vi "CollectData.vi"(7 "LabVIEW Web Service Request":refnum<class "Web Request.lvclass">) -> ()   [LabVIEW 2017]
uses:
  <vilib>/wsapi/Web Request.lvclass
  <vilib>/rvi/interface/nirviOpenFPGA/nirviOpenFPGA.xnode
  <vilib>/rvi/interface/nirviCloseFPGA/nirviCloseFPGA.xnode
  <vilib>/FPGAPlugInAG/Dynamic/niLvFpga_Close_Dynamic.vi
  <vilib>/rvi/interface/nirviReadWriteControl/nirviReadWriteControl.xnode
  NiFpgaLv.dll
  <vilib>/Utility/error.llb/Error Cluster From Error Code.vi
  <vilib>/rvi/interface/Simulation/niFpgaSimulationCallBeginRW.vi
  <vilib>/rvi/errors/niLvFpgaAdjustHostInterfaceError.vi
  It Just Works/LabVIEW/FPGA Bitfiles/sbRIOtest_FPGATarget2_DAQgenV4_A5bgOiEgHgk.lvbitx
  It Just Works/LabVIEW/DAQgenV4.vi
  <vilib>/FPGAPlugInAG/sbRIO-9633/niLvFpga_Open_sbRIO-9633.vi
  <vilib>/rvi/interface/common/dynamic/niFpgaDynamicAddResources.vi
panel:
  # "Use the Web Service Request input terminal to call the VIs on the Web Services palette. Do not remove it from the connector pane unless you don't need access to the palette."
  # "Each additional control wired to the connector pane will be available as an input in the URL. To include an indicator in terminal-mode output (the default setting), it must also be wired to the connector pane."
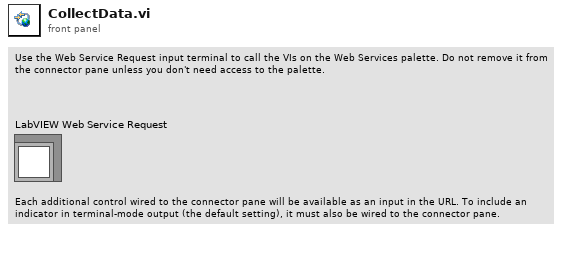
[diagram p1: front panel]
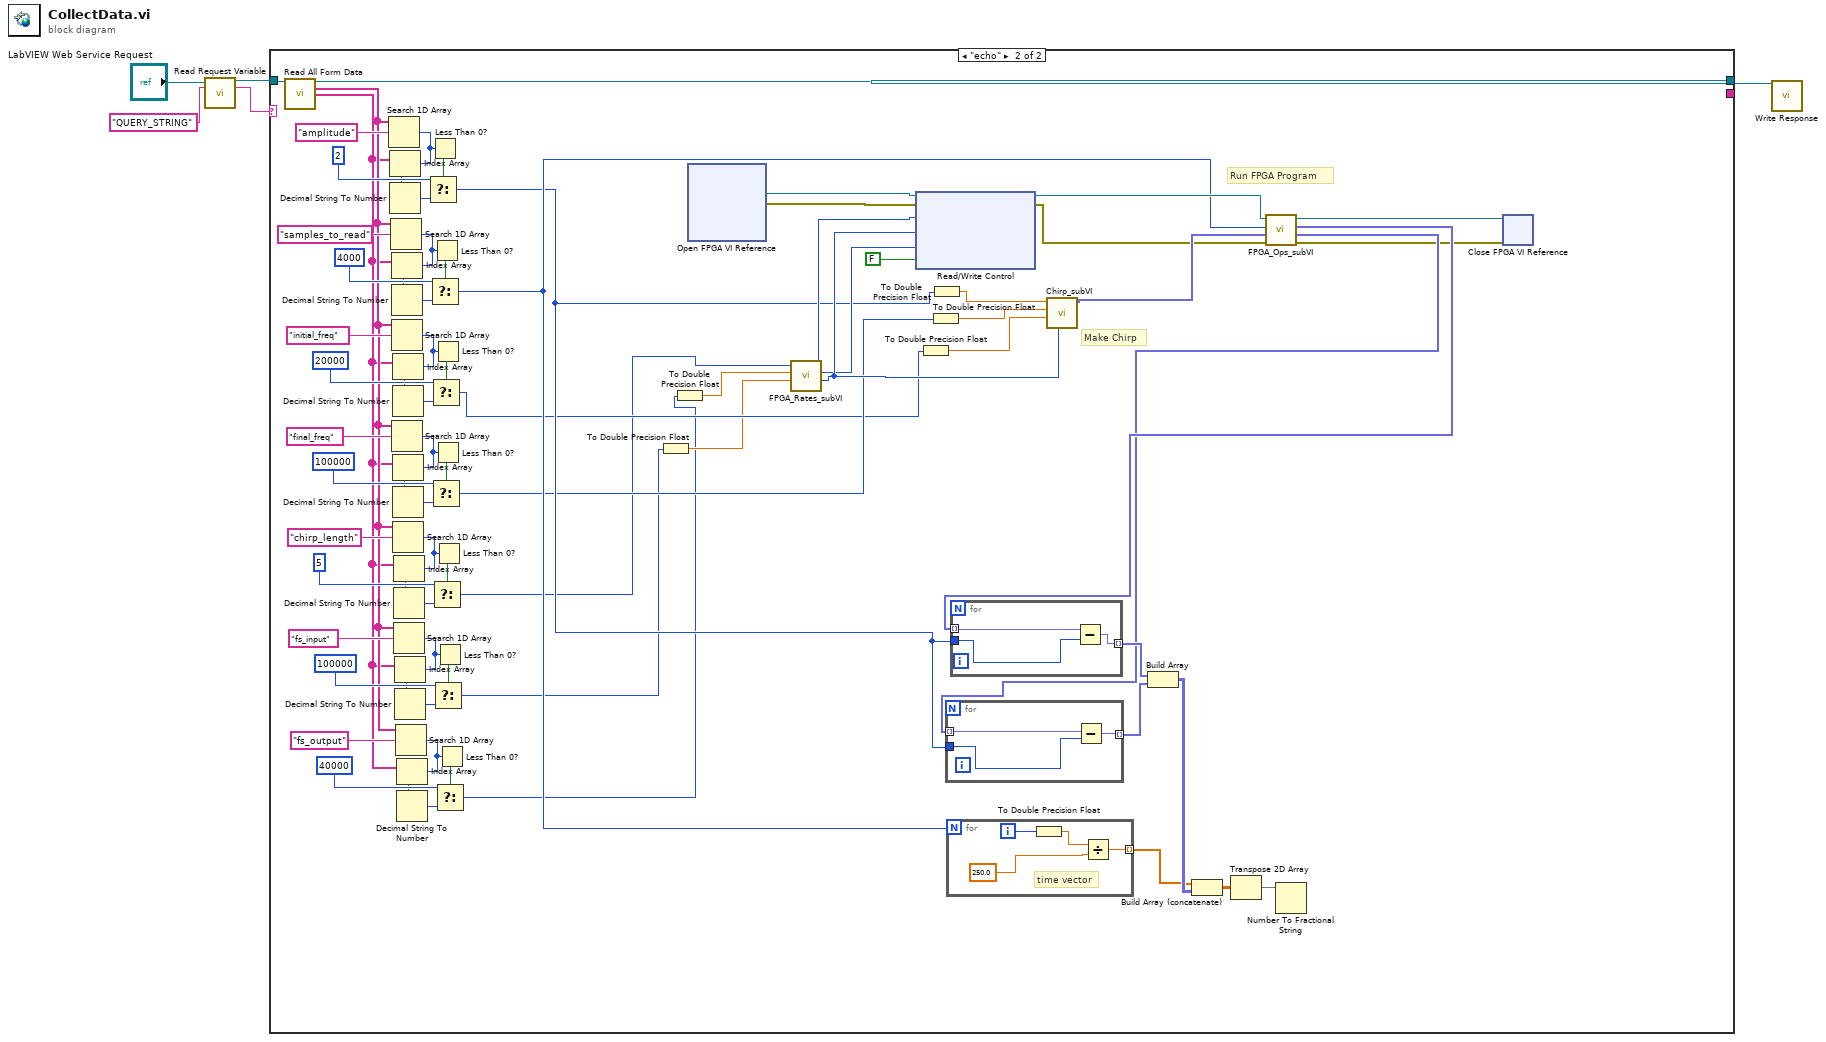
[diagram p0: block diagram]
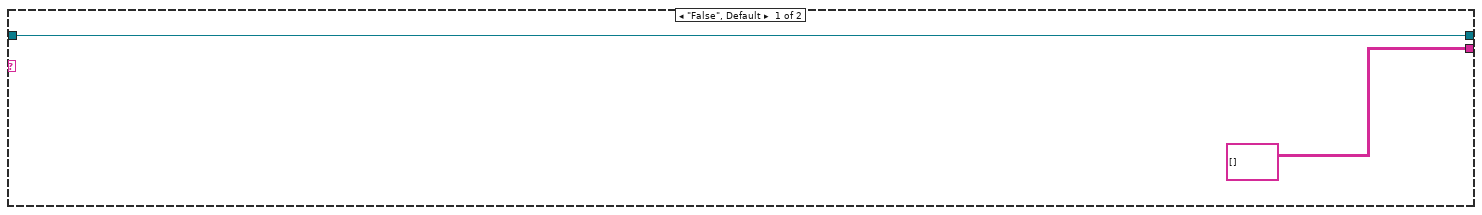
[diagram p2: hidden frame]
diagram:
  n1 = call <vilib>:"Read Request Variable.vi"("LabVIEW Web Service Request"="LabVIEW Web Service Request", "variable name"="QUERY_STRING") -> ("LabVIEW Web Service Request out"=w2:refnum<class "Web Request.lvclass">, "value"=w3:string)  [unwired: 11 in, 1 out]
  n2 = case shown="\"echo\"" w3 {
    tunnel: w2 -> [w7 w85]
    tunnel: [w7 w84] -> w1
    tunnel: [string[][] [] _] -> _
    frame "False", Default {
    }
    frame "echo" {
      # "Run FPGA Program"
      # "Make Chirp"
      n3 = call <vilib>:"Read All Form Data.vi"("LabVIEW Web Service Request"=w85) -> ("LabVIEW Web Service Request out"=w84:refnum<class "Web Request.lvclass">, "Key"=w13:string[], "Value"=w12:string[])  [unwired: 10 in, 2 out]
      n4 = Search 1D Array(1D array=w13, element="amplitude") -> (index of element=w79:i32)  [unwired: 1 in]
      n5 = Index Array(array=w12, index=w79) -> (element=w80:string)
      n6 = Decimal String To Number(string=w80) -> (number=w78:i32)  [unwired: 2 in, 1 out]
      n7 = Search 1D Array(1D array=w13, element="samples_to_read") -> (index of element=w73:i32)  [unwired: 1 in]
      n8 = Index Array(array=w12, index=w73) -> (element=w74:string)
      n9 = Decimal String To Number(string=w74) -> (number=w72:i32)  [unwired: 2 in, 1 out]
      n10 = Search 1D Array(1D array=w13, element="initial_freq") -> (index of element=w67:i32)  [unwired: 1 in]
      n11 = Search 1D Array(1D array=w13, element="final_freq") -> (index of element=w38:i32)  [unwired: 1 in]
      n12 = Index Array(array=w12, index=w67) -> (element=w68:string)
      n13 = Decimal String To Number(string=w68) -> (number=w66:i32)  [unwired: 2 in, 1 out]
      n14 = Index Array(array=w12, index=w38) -> (element=w39:string)
      n15 = Decimal String To Number(string=w39) -> (number=w37:i32)  [unwired: 2 in, 1 out]
      n16 = Search 1D Array(1D array=w13, element="chirp_length") -> (index of element=w28:i32)  [unwired: 1 in]
      n17 = Index Array(array=w12, index=w28) -> (element=w29:string)
      n18 = Decimal String To Number(string=w29) -> (number=w27:i32)  [unwired: 2 in, 1 out]
      n19 = Search 1D Array(1D array=w13, element="fs_input") -> (index of element=w21:i32)  [unwired: 1 in]
      n20 = Index Array(array=w12, index=w21) -> (element=w22:string)
      n21 = Decimal String To Number(string=w22) -> (number=w20:i32)  [unwired: 2 in, 1 out]
      n22 = Search 1D Array(1D array=w13, element="fs_output") -> (index of element=w15:i32)  [unwired: 1 in]
      n23 = Index Array(array=w12, index=w15) -> (element=w16:string)
      n24 = Decimal String To Number(string=w16) -> (number=w14:i32)  [unwired: 2 in, 1 out]
      n25 = Less Than 0?(x=w79) -> (x < 0?=w83:bool)
      n26 = Select(t=2, s=w83, f=w78) -> (s? t:f=w44:i32)
      n27 = Less Than 0?(x=w73) -> (x < 0?=w77:bool)
      n28 = Select(t=4000, s=w77, f=w72) -> (s? t:f=w46:i32)
      n29 = Less Than 0?(x=w67) -> (x < 0?=w71:bool)
      n30 = Select(t=20000, s=w71, f=w66) -> (s? t:f=w33:i32)
      n31 = Less Than 0?(x=w38) -> (x < 0?=w42:bool)
      n32 = Select(t=100000, s=w42, f=w37) -> (s? t:f=w35:i32)
      n33 = Less Than 0?(x=w28) -> (x < 0?=w32:bool)
      n34 = Select(t=5, s=w32, f=w27) -> (s? t:f=w26:i32)
      n35 = Less Than 0?(x=w21) -> (x < 0?=w25:bool)
      n36 = Select(t=100000, s=w25, f=w20) -> (s? t:f=w10:i32)
      n37 = Less Than 0?(x=w15) -> (x < 0?=w19:bool)
      n38 = Select(t=40000, s=w19, f=w14) -> (s? t:f=w8:i32)
      n39 = To Double Precision Float(number=w10) -> (double precision float=w11:dbl)
      n40 = To Double Precision Float(number=w8) -> (double precision float=w9:dbl)
      n41 = xnode "Open FPGA VI Reference"() -> ("FPGA VI Reference Out"=w59:refnum<k20>, "error out"=w62:errorcluster)  [unwired: 2 in]
      n42 = call "FPGA_Rates_subVI.vi"("Fs In (Hz)"=w11, "Fs Out (Hz)"=w9, "Chirp Len (ms)"=w26) -> ("# Output Samples"=w65:i16, "Input Ticks (ticks/S)"=w60:u32, "Output Ticks (ticks/S)"=w58:u32)  [unwired: 5 in, 1 out]
      n43 = xnode "Read/Write Control"("FPGA VI Reference In"=w59, "error in"=w62, "Sampling Rate (Hz)"=w58, "# Samples"=w65, "Count(Ticks)"=w60, "Wavegen!"=FALSE) -> ("FPGA VI Reference Out"=w61:refnum<k20>, "error out"=w63:errorcluster)
      n44 = To Double Precision Float(number=w33) -> (double precision float=w34:dbl)
      n45 = To Double Precision Float(number=w35) -> (double precision float=w36:dbl)
      n46 = To Double Precision Float(number=w44) -> (double precision float=w43:dbl)
      n47 = for {
        N: w46 -> [_]
        tunnel: [w93] -> w52 mode=indexing
        i -> [w95]
        # "time vector"
        n48 = To Double Precision Float(number=w95) -> (double precision float=w94:dbl)
        n49 = Divide(x=w94, y=250.0) -> (x/y=w93:dbl)
      }
      n50 = call "Chirp_subVI.vi"("# Output Samples"=w65, "Initial Frequency (Hz)"=w34, "Final Frequency (Hz)"=w36, "Amplitude (V)"=w43) -> ("Chirp"=w64:fxp<+,16,3>[])  [unwired: 7 in]
      n51 = call "FPGA_Ops_subVI.vi"("error in (no error)"=w63, "Chirp"=w64, "Samples to Read"=w46, "FPGA VI Reference Out"=w61) -> ("error out"=w45:errorcluster, "Data B"=w48:fxp<+,16,3>[], "Data A"=w49:fxp<+,16,3>[], "Refnum out"=w57:refnum<k20>)  [unwired: 4 in]
      n52 = for {
        tunnel: w48 -> [w91] mode=indexing
        tunnel: [w90] -> w50 mode=indexing
        tunnel: w44 -> [w89]
        n53 = Subtract(x=w91, y=w89) -> (x-y=w90:fxp<+/-,46,33>)
      }
      n54 = for {
        tunnel: w49 -> [w88] mode=indexing
        tunnel: [w87] -> w51 mode=indexing
        tunnel: w44 -> [w86]
        n55 = Subtract(x=w88, y=w86) -> (x-y=w87:fxp<+/-,46,33>)
      }
      n56 = Build Array(w51, w50) -> (w55:fxp<+/-,46,33>[][])
      n57 = Build Array (concatenate)(w52, w55) -> (w54:dbl[][])
      n58 = Transpose 2D Array(2D array=w54) -> (transposed array=w53:dbl[][])
      n59 = Number To Fractional String(number=w53) -> (F-format string=w47:string[][])  [unwired: 3 in]
      n60 = xnode "Close FPGA VI Reference"("FPGA VI Reference In"=w57, "error in"=w45) -> ()  [unwired: 1 out]
    }
  }
  n61 = call <vilib>:"Write Response.vi"("LabVIEW Web Service Request"=w1) -> ()  [unwired: 13 in, 2 out]
